vi "Size.vi"(7 "VI":refnum<vi>, 8 "Error":errorcluster, 9 "WkSpace":T1, 11 "GObject_FPSZ":refnum<class "GObject_FPSZ.lvclass">) -> (0 "Error Out":errorcluster, 3 "GObject_FPSZ Out":refnum<class "GObject_FPSZ.lvclass">, 5 "VI Out":refnum<vi>)   [LabVIEW 2016, in "GObject_FPSZ.lvclass"]
uses:
  GObject_FPSZ.lvclass
  E:/~Data/FRC/Magic Trident/Code/UI LED Build file Interface/Utility/Universal Utility/FP/FPClass/(FPSZ)/(FPSZ).lvclass
  <vilib>/Utility/miscctls.llb/LVRectTypeDef.ctl
  GObject_FPSZ.lvclass/GObject_FPSZ.ctl
  (FPSZ).lvclass
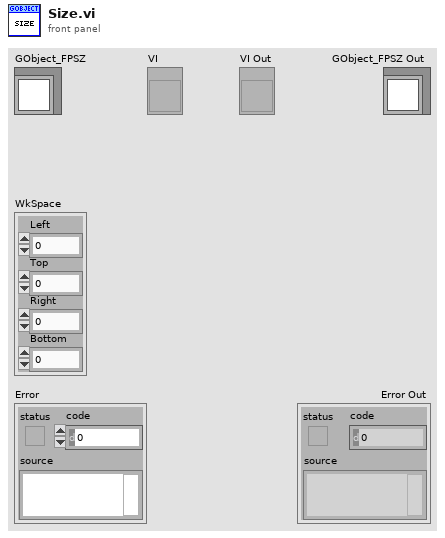
[diagram p1: front panel]
types:
  T1 = typedef "LVRectTypeDef.ctl" = cluster{"Left":i16, "Top":i16, "Right":i16, "Bottom":i16}
  T2 = typedef "LVBoundsTypeDef.ctl" = cluster{"Width":u32, "Height":u32}
  T3 = typedef "LVPositionTypeDef.ctl" = cluster{"Left":i32, "Top":i32}
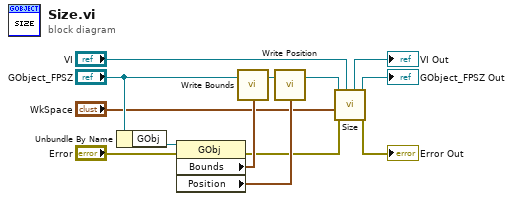
[diagram p0: block diagram]
diagram:
  n1 = Unbundle By Name("GObject_FPSZ") -> ("GObj"=w9:refnum<vi>)
  n2 = property class="GObj"(reference=w9, error in="Error") -> (error out=w2:errorcluster, "Bounds"=w5:T2, "Position"=w4:T3)  [unwired: 1 out]
  n3 = call "Write Bounds.vi"("(FPSZ)"="GObject_FPSZ", "Bounds"=w5) -> ("(FPSZ) Out"=w7:refnum<class "GObject_FPSZ.lvclass">)  [unwired: 3 in]
  n4 = call "Write Position.vi"("(FPSZ)"=w7, "Position"=w4) -> ("(FPSZ) Out"=w6:refnum<class "GObject_FPSZ.lvclass">)  [unwired: 3 in]
  n5 = call-parent "Size.vi"("VI"="VI", "Error"=w2, "WkSpace"="WkSpace", "(FPSZ)"=w6) -> ("Error Out"=→"Error Out":errorcluster, "(FPSZ) Out"=→"GObject_FPSZ Out":refnum<class "GObject_FPSZ.lvclass">, "VI Out"=→"VI Out":refnum<vi>)  [unwired: 5 in]
